vi "Test Arduino Temperature Controller.vi"() -> ()   [LabVIEW 2018]
panel:
  out "IDN":string
  out "read buffer 3":string
  out "T2":string
  in  "Serial Settings:Baud Rate":u32=9600
  out "T1":string
  in  "VISA resource name":refnum<visa-resource-name>
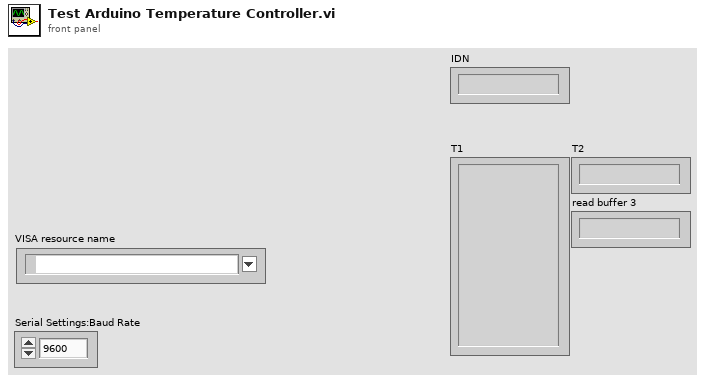
[diagram p1: front panel]
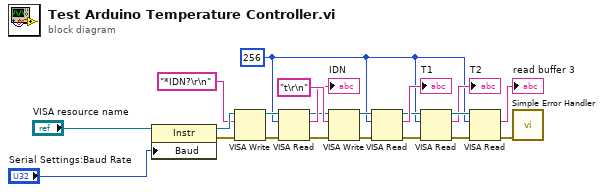
[diagram p0: block diagram]
diagram:
  w5 = u32 256 ("byte count")
  n1 = property class="Instr"(reference="VISA resource name", "Baud"="Serial Settings:Baud Rate") -> (reference out=w9:refnum<visa-resource-name>, error out=w10:errorcluster)  [unwired: 1 in]
  n2 = VISA Write(VISA resource name=w9, write buffer="*IDN?\r\n", error in (no error)=w10) -> (VISA resource name out=w6:refnum<visa-resource-name>, error out=w7:errorcluster)  [unwired: 1 out]
  n3 = VISA Read(VISA resource name=w6, byte count=w5, error in (no error)=w7) -> (VISA resource name out=w3:refnum<visa-resource-name>, read buffer=→"IDN":string, error out=w2:errorcluster)  [unwired: 1 out]
  n4 = VISA Write(VISA resource name=w3, write buffer="t\r\n", error in (no error)=w2) -> (VISA resource name out=w20:refnum<visa-resource-name>, error out=w19:errorcluster)  [unwired: 1 out]
  n5 = VISA Read(VISA resource name=w20, byte count=w5, error in (no error)=w19) -> (VISA resource name out=w16:refnum<visa-resource-name>, read buffer=→"T1":string, error out=w14:errorcluster)  [unwired: 1 out]
  n6 = VISA Read(VISA resource name=w16, byte count=w5, error in (no error)=w14) -> (VISA resource name out=w15:refnum<visa-resource-name>, read buffer=→"T2":string, error out=w13:errorcluster)  [unwired: 1 out]
  n7 = VISA Read(VISA resource name=w15, byte count=w5, error in (no error)=w13) -> (read buffer=→"read buffer 3":string, error out=w1:errorcluster)  [unwired: 2 out]
  n8 = call <vilib>:"Simple Error Handler.vi"("error in (no error)"=w1) -> ()  [unwired: 4 in, 5 out]
